vi "event.vi"() -> ()   [LabVIEW 2020]
panel:
  out "String":string
  in  "stop":bool
  in  "B":bool
  in  "A":bool
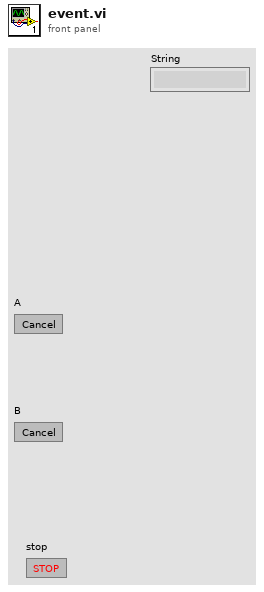
[diagram p1: front panel]
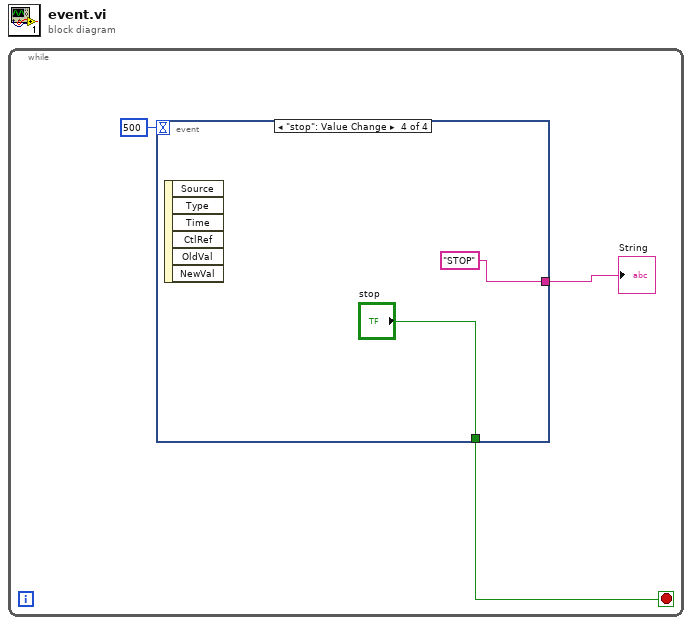
[diagram p0: block diagram]
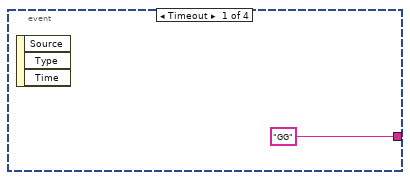
[diagram p2: hidden frame]
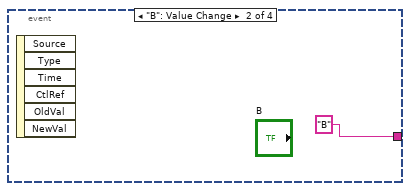
[diagram p3: hidden frame]
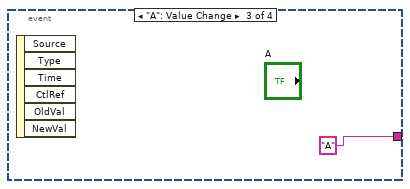
[diagram p4: hidden frame]
diagram:
  n1 = while {
    stop <- w1 stop-if-true
    n2 = event shown="[3] \"stop\": Value Change" {
      selector: _ -> [_ _ _ _]
      dyn-events: _ -> [_ _ _ _]
      timeout: 500 -> [_ _ _ _]
      tunnel: ["GG" "B" "A" "STOP"] -> w2
      tunnel: [_ _ _ "stop"] -> w1
      event Timeout {
        n3 = event-data() -> ()  [unwired: 1 in, 3 out]
      }
      event "B": Value Change {
        n4 = event-data() -> ()  [unwired: 1 in, 6 out]
      }
      event "A": Value Change {
        n5 = event-data() -> ()  [unwired: 1 in, 6 out]
      }
      event "stop": Value Change {
        n6 = event-data() -> ()  [unwired: 1 in, 6 out]
      }
    }
    "String" <- w2
  }
